vi "SendValuesOfAnglesVIASerial.vi"(8 "error in (no error)":errorcluster, 10 "Data":T1(array[cluster]), 11 "VISA Refnum in":refnum<visa-resource-name>) -> (0 "error out":errorcluster, 3 "VISA Refnum out":refnum<visa-resource-name>)   [LabVIEW 2014, in "Manipulator.lvclass"]
uses:
  Manipulator.lvclass
  <vilib>/Instr/_visa.llb/VISA Flush IO Buffer Mask.ctl
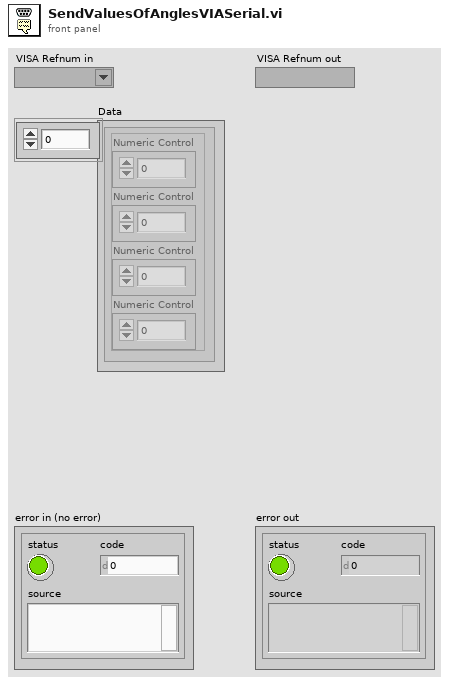
[diagram p1: front panel]
types:
  T1 = cluster{"Numeric Control":dbl, "Numeric Control":dbl, "Numeric Control":dbl, "Numeric Control":dbl}[]
  T2 = cluster{"Numeric Control":dbl, "Numeric Control":dbl, "Numeric Control":dbl, "Numeric Control":dbl}
  T3 = typedef "VISA Flush IO Buffer Mask.ctl" = u16
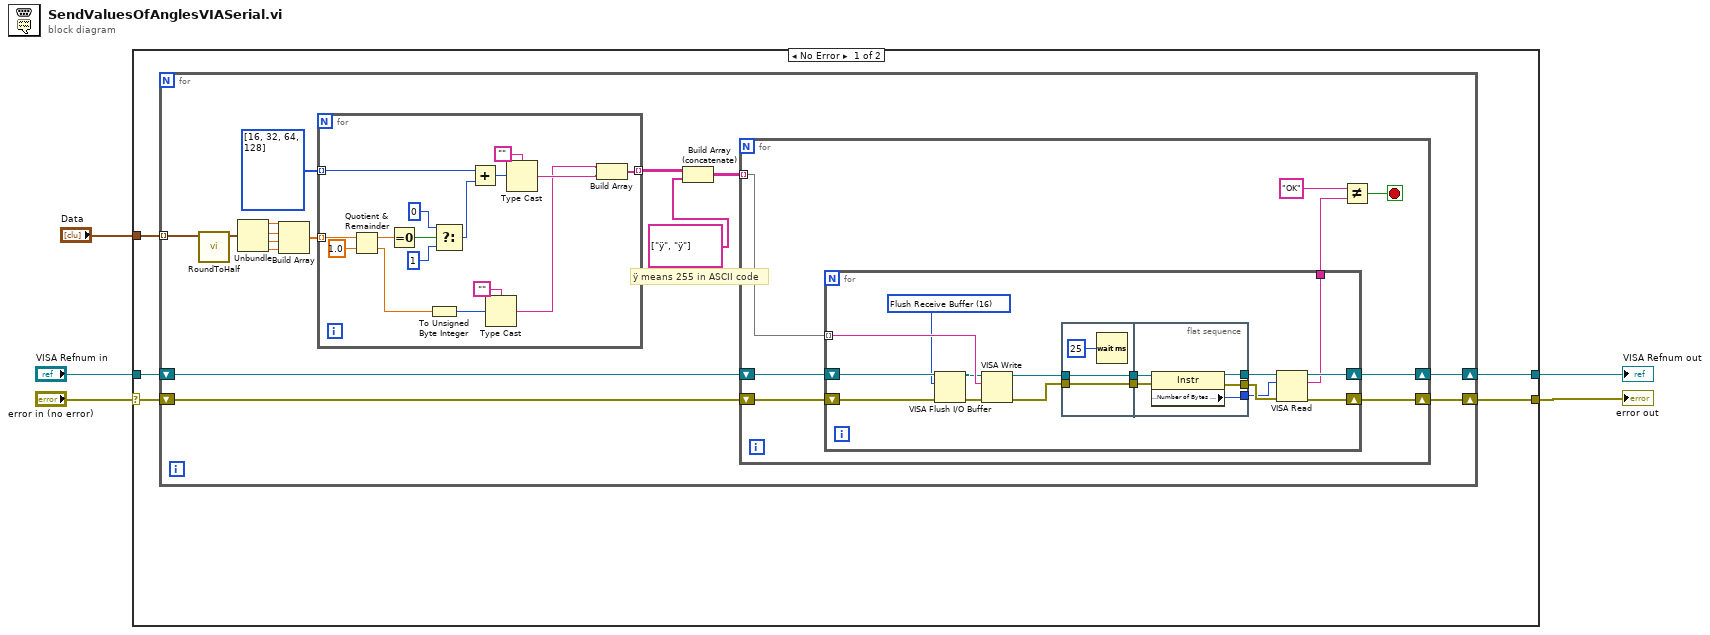
[diagram p0: block diagram]
diagram:
  n1 = case shown="No Error" "error in (no error)" {
    selector: "error in (no error)" -> [w6 w74]
    tunnel: [w10 w75] -> w1
    tunnel: "VISA Refnum in" -> [w9 w75]
    tunnel: "Data" -> [w8 _]
    tunnel: [w7 w74] -> w4
    frame No Error {
      n2 = for {
        shift-right: [w24] -> w10
        shift-left: w9 -> [w23]
        shift-right: [w25] -> w7
        shift-left: w6 -> [w22]
        tunnel: w8 -> [w14] mode=indexing
        # "ÿ means 255 in ASCII code"
        n3 = call "RoundToHalf.vi"("Cluster in"=w14) -> ("Cluster out"=w21:T2)  [unwired: 10 in]
        n4 = Unbundle(w21) -> ("Numeric Control"=w20:dbl, "Numeric Control"=w17:dbl, "Numeric Control"=w18:dbl, "Numeric Control"=w19:dbl)
        n5 = Build Array(w20, w17, w18, w19) -> (w16:dbl[])
        n6 = for {
          tunnel: w16 -> [w41] mode=indexing
          tunnel: u8[] [16, 32, 64, 128] -> [w31] mode=indexing
          tunnel: [w28] -> w12 mode=indexing
          n7 = Quotient & Remainder(x=w41, y=1.0) -> (x-y*floor(x/y)=w38:dbl, floor(x/y)=w37:dbl)
          n8 = Equal To 0?(x=w38) -> (x = 0?=w39:bool)
          n9 = To Unsigned Byte Integer(number=w37) -> (unsigned 8bit integer=w36:u8)
          n10 = Select(t=u8 0, s=w39, f=u8 1) -> (s? t:f=w30:u8)
          n11 = Add(x=w31, y=w30) -> (x+y=w32:u8)
          n12 = Type Cast(type="", x=w36) -> (*(type *) &x=w26:string)
          n13 = Type Cast(type="", x=w32) -> (*(type *) &x=w27:string)
          n14 = Build Array(w26, w27) -> (w28:string[])
        }
        n15 = Build Array (concatenate)(w12, string[] ["ÿ", "ÿ"]) -> (w11:string[][])
        n16 = for {
          shift-right: [w47] -> w24
          shift-left: w23 -> [w49]
          shift-right: [w46] -> w25
          shift-left: w22 -> [w48]
          tunnel: w11 -> [w42] mode=indexing
          stop <- w45 stop-if-true
          n17 = for {
            tunnel: [w60] -> w43
            shift-right: [w62] -> w47
            shift-left: w49 -> [w54]
            shift-right: [w61] -> w46
            shift-left: w48 -> [w52]
            tunnel: w42 -> [w55] mode=indexing
            w50 = T3 16 items=["Flush Receive Buffer"=16, "Write Transmit Buffer to Device"=32, "Flush Receive Buffer (No I/O)"=64, "Flush Transmit Buffer"=128] ("Mask")
            n18 = VISA Flush I/O Buffer(VISA resource name=w54, mask (16)=w50, error in (no error)=w52) -> (VISA resource name out=w53:refnum<visa-resource-name>, error out=w51:errorcluster)
            n19 = VISA Write(VISA resource name=w53, write buffer=w55, error in (no error)=w51) -> (VISA resource name out=w56:refnum<visa-resource-name>, error out=w63:errorcluster)  [unwired: 1 out]
            n20 = flat-sequence {
              tunnel: w63 -> [w67]
              tunnel: w56 -> [w68]
              tunnel: [w68] -> w65
              tunnel: [w67] -> w64
              tunnel: w65 -> [w73]
              tunnel: w64 -> [w72]
              tunnel: [w71] -> w57
              tunnel: [w70] -> w58
              tunnel: [w69] -> w59
              frame #0 {
                n21 = Wait (ms)(milliseconds to wait=u32 25) -> ()  [unwired: 1 out]
              }
              frame #1 {
                n22 = property class="Instr"(reference=w73, error in=w72) -> (reference out=w69:refnum<visa-resource-name>, error out=w70:errorcluster, "Serial Settings:Number of Bytes at Serial Port"=w71:u32)
              }
            }
            n23 = VISA Read(VISA resource name=w59, byte count=w57, error in (no error)=w58) -> (VISA resource name out=w62:refnum<visa-resource-name>, read buffer=w60:string, error out=w61:errorcluster)  [unwired: 1 out]
          }
          n24 = Not Equal?(x="OK", y=w43) -> (x != y?=w45:bool)
        }
      }
    }
    frame Error {
    }
  }
  "error out" <- w4
  "VISA Refnum out" <- w1
